vi "示波器.vi"() -> ()   [LabVIEW 2020]
panel:
  out "data":dynamicdata(graph)
  in  "rate":dbl=10000.0
  in  "number of samples":i32=1000
  in  "stop":bool
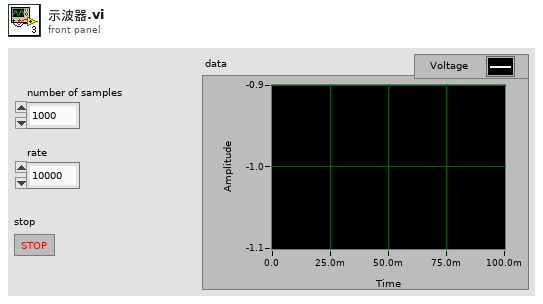
[diagram p1: front panel]
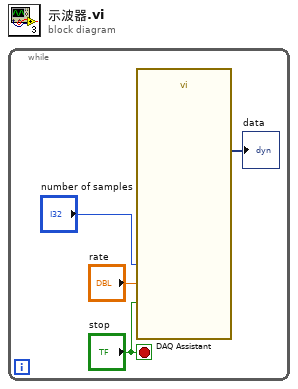
[diagram p0: block diagram]
diagram:
  n1 = while {
    stop <- "stop" stop-if-true
    n2 = call "DAQ Assistant"("rate"="rate", "number of samples"="number of samples", "stop (F)"="stop") -> ("data"=→"data":dynamicdata)  [unwired: 13 in, 3 out]
  }
